vi "ROS_Service_Setup.vi"(3 "Specs":T3={"Server"="", "Node"="/labview", "Server Port"=5000, "URI (Subsc)"="", "connection"=refnum, "Direction"=enum."Node"}, 4 "Msg to Send":string, 5 "Requests In":T1(array[cluster])) -> (0 "error out":errorcluster, 1 "Reply":string, 2 "Requests Out":T1(array[cluster]))   [LabVIEW 2013]
doc: "Creates and sends the connection header and message to a service provider. Implemented in the background server."
uses:
  SubVIs/_ROSDirection.ctl
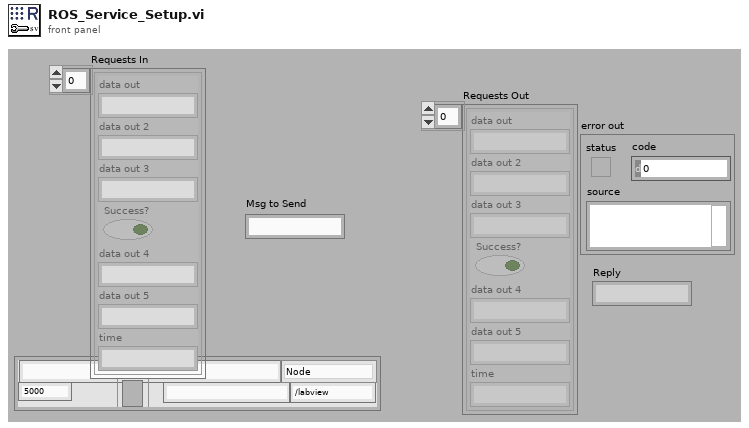
[diagram p1: front panel]
types:
  T1 = cluster{"data out":string, "data out 2":string, "data out 3":string, "Success?":bool, "data out 4":string, "data out 5":string, "time":string}[]
  T2 = typedef "_ROSDirection.ctl" = enum16{"Node", "Publisher", "Subscriber", "Service Client"}
  T3 = cluster{"Server":string, "Node":string, "Server Port":u32, "URI (Subsc)":string, "connection":refnum<k5>, "Direction":T2}
  T4 = cluster{"data out":string, "data out 2":string, "data out 3":string, "Success?":bool, "data out 4":string, "data out 5":string, "time":string}
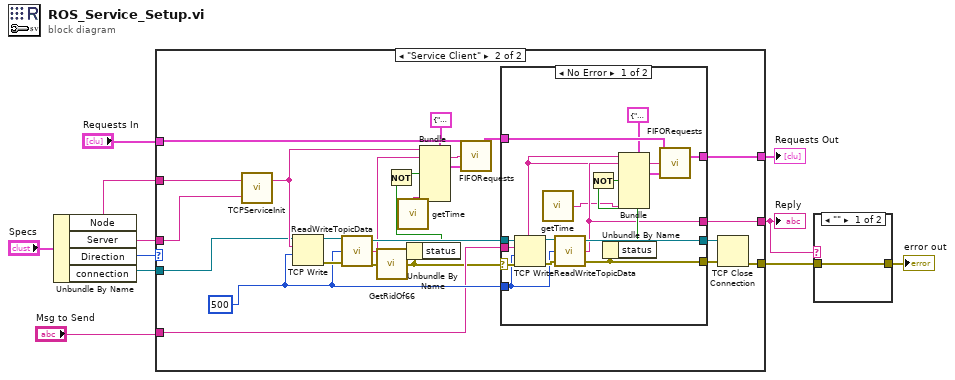
[diagram p0: block diagram]
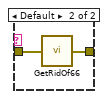
[diagram p2: hidden frame]
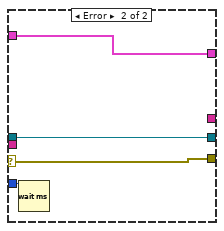
[diagram p4: hidden frame]
diagram:
  n1 = Unbundle By Name("Specs") -> ("Node"=w9:string, "Server"=w8:string, "Direction"=w10:T2, "connection"=w1:refnum<k5>)
  n2 = case shown="\"Service Client\"" w10 {
    tunnel: w9 -> [_ w29]
    tunnel: w8 -> [_ w28]
    tunnel: "Requests In" -> [w12 w27]
    tunnel: [w12 w20] -> w6
    tunnel: [_ w22] -> w3
    tunnel: "Msg to Send" -> [_ w19]
    tunnel: [_ w18] -> w4
    tunnel: w1 -> [_ w17]
    frame Default {
    }
    frame "Service Client" {
      w30 = 500 ("timeout ms (60000)")
      n3 = call "TCPServiceInit.vi"("topic"=w28, "callerID"=w29) -> ("TCP ROS Reply"=w33:string)  [unwired: 1 out]
      n4 = TCP Write(connection ID=w17, data in=w33, 9:w30) -> (connection ID out=w36:refnum<k5>, error out=w35:errorcluster)  [unwired: 1 in, 1 out]
      n5 = call "ReadWriteTopicData.vi"("error in (no error)"=w35, "timeout ms (1000)"=w30, "connection ID in"=w36) -> ("error out"=w16:errorcluster, "data out"=w31:string, "connection ID out"=w34:refnum<k5>)
      n6 = call "GetRidOf66.vi"("error in (no error)"=w16) -> ("error out"=w15:errorcluster)
      n7 = call "getTime.vi"() -> ("Current Time"=w13:string)  [unwired: 1 in]
      n8 = Unbundle By Name(w15) -> ("status"=w25:bool)
      n9 = Not(x=w25) -> (.not. x?=w24:bool)
      n10 = Bundle(cluster=T4 {"data out"="", "data out 2"="", "data out 3"="", "Success?"=FALSE, "data out 4"="", "data out 5"="", "time"=""}, "data out"=w33, "data out 2"=w31, "Success?"=w24, "time"=w13) -> (w32:T4)  [unwired: 3 in]
      n11 = call "FIFORequests.vi"("New One"=w32, "data out"=w31, "Requests In"=w27) -> ("Requests Out"=w21:T1)
      n12 = case shown="No Error" w15 {
        selector: w15 -> [w48 w54]
        tunnel: w34 -> [w50 w55]
        tunnel: w30 -> [w39 w56]
        tunnel: [w49 w55] -> w26
        tunnel: [w44 w54] -> w23
        tunnel: w21 -> [w46 w53]
        tunnel: [w45 w53] -> w20
        tunnel: w19 -> [w40 _]
        tunnel: [w41 _] -> w18
        frame No Error {
          n13 = TCP Write(connection ID=w50, data in=w40, error in (no error)=w48, 9:w39) -> (connection ID out=w52:refnum<k5>, error out=w51:errorcluster)  [unwired: 1 out]
          n14 = call "getTime.vi"() -> ("Current Time"=w37:string)  [unwired: 1 in]
          n15 = call "ReadWriteTopicData.vi"("error in (no error)"=w51, "timeout ms (1000)"=w39, "connection ID in"=w52) -> ("error out"=w44:errorcluster, "data out"=w41:string, "connection ID out"=w49:refnum<k5>)
          n16 = Unbundle By Name(w44) -> ("status"=w43:bool)
          n17 = Not(x=w43) -> (.not. x?=w42:bool)
          n18 = Bundle(cluster=T4 {"data out"="", "data out 2"="", "data out 3"="", "Success?"=FALSE, "data out 4"="", "data out 5"="", "time"=""}, "data out"=w40, "data out 2"=w41, "Success?"=w42, "time"=w37) -> (w47:T4)  [unwired: 3 in]
          n19 = call "FIFORequests.vi"("New One"=w47, "data out"=w40, "Requests In"=w46) -> ("Requests Out"=w45:T1)
        }
        frame Error {
          n20 = Wait (ms)(milliseconds to wait=w56) -> ()  [unwired: 1 out]
        }
      }
      n21 = TCP Close Connection(connection ID=w26, error in (no error)=w23) -> (error out=w22:errorcluster)  [unwired: 1 in, 1 out]
    }
  }
  "Requests Out" <- w6
  "Reply" <- w4
  n22 = case shown="\"\"" w4 {
    tunnel: w3 -> [w57 w59]
    tunnel: [w57 w58] -> w2
    frame "" {
    }
    frame Default {
      n23 = call "GetRidOf66.vi"("error in (no error)"=w59) -> ("error out"=w58:errorcluster)
    }
  }
  "error out" <- w2
